vi "Read headers.vi"(8 "error in (no error)":errorcluster, 11 "httpResponse in":refnum<class "httpResponse.lvclass">) -> (0 "error out":errorcluster, 2 "headers":string, 3 "httpResponse out":refnum<class "httpResponse.lvclass">)   [LabVIEW 2020, in "httpClient.lvlib" / "httpResponse.lvclass"]
uses:
  httpResponse.lvclass
  httpResponse.lvclass/httpResponse.ctl
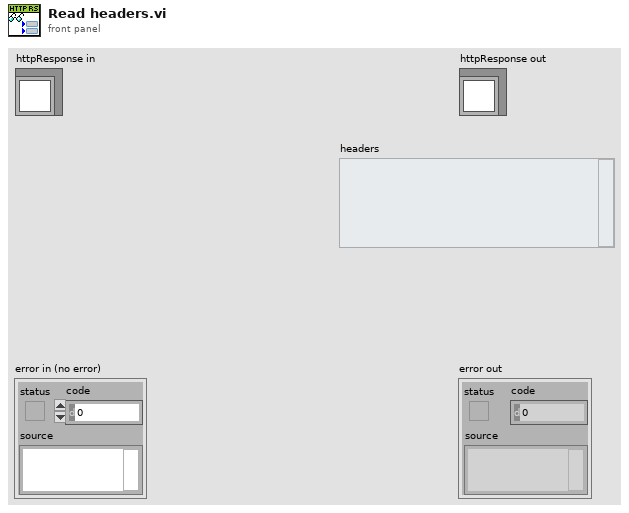
[diagram p1: front panel]
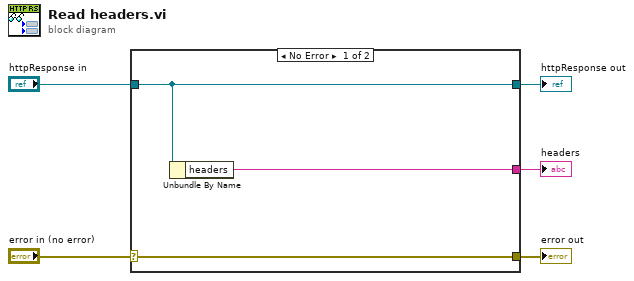
[diagram p0: block diagram]
diagram:
  n1 = case shown="No Error" "error in (no error)" {
    selector: "error in (no error)" -> [w8 w9]
    tunnel: [w8 w9] -> w4
    tunnel: [w7 w10] -> w2
    tunnel: "httpResponse in" -> [w7 w10]
    tunnel: [w6 _] -> w1
    frame No Error {
      n2 = Unbundle By Name(w7) -> ("headers"=w6:string)
    }
    frame Error {
    }
  }
  "error out" <- w4
  "httpResponse out" <- w2
  "headers" <- w1
